vi "Add Stage Section.vi"(8 "error in (no error)":errorcluster, 10 "Analysis Options":T1={"Pull In Time"=TRUE, "Pull In Max Current"=TRUE, "Pull In Max Voltage"=TRUE, "Pull In Min Voltage"=TRUE, "Pull In Avg Voltage"=TRUE, "Hold In Time"=TRUE, "Hold In Max Current"=TRUE, "Hold In Min Current"=TRUE, "Hold In Avg Current"=TRUE, "Hold In Max Voltage"=TRUE, "Hold In Min Voltage"=TRUE, "Hold In Avg Max Voltage"=TRUE, "Hold In Avg Min Voltage"=TRUE, "Off Time"=TRUE, "Off Stage Max Current"=TRUE, "Off Stage Min Current"=TRUE, "Off Stage Avg Current"=TRUE, "Off Stage Max Voltage"=TRUE, "Off Stage Min Voltage"=TRUE, "Off Stage Avg Voltage"=TRUE, "Total Voltage Pulses"=TRUE, "Total Stage Time"=TRUE}, 11 "Shot Section reference in":T2=18446744073709551615 format="%.0x") -> (0 "error out":errorcluster, 3 "Shot Section reference out":T2=18446744073709551615 format="%.0x")   [LabVIEW 2015, in "Fuel Injector Analysis Addon System Explorer.lvlib"]
uses:
  Fuel Injector Analysis Addon System Explorer.lvlib
  <vilib>/NI Veristand/Custom Device API/Custom Device Item Ref.ctl
  Shared/Types/Analysis.Channels.Select.ctl
  <vilib>/NI Veristand/Custom Device API/Custom Device Channel.ctl
  <vilib>/NI Veristand/Custom Device API/Custom Device Channel Type.ctl
  Shared/Constants.vi
  Shared/Fuel Injector Analysis Addon Shared.lvlib
  <vilib>/NI Veristand/Custom Device API/Custom Device API.lvlib
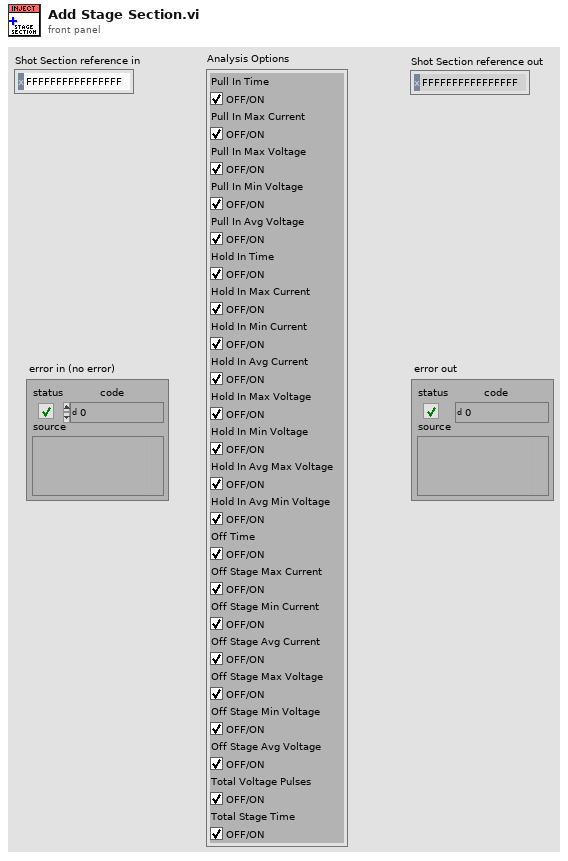
[diagram p1: front panel]
types:
  T1 = typedef "Fuel Injector Analysis Addon Shared.lvlib/Analysis.Channels.Select.ctl" = cluster{"Pull In Time":bool, "Pull In Max Current":bool, "Pull In Max Voltage":bool, "Pull In Min Voltage":bool, "Pull In Avg Voltage":bool, "Hold In Time":bool, "Hold In Max Current":bool, "Hold In Min Current":bool, "Hold In Avg Current":bool, "Hold In Max Voltage":bool, "Hold In Min Voltage":bool, "Hold In Avg Max Voltage":bool, "Hold In Avg Min Voltage":bool, "Off Time":bool, "Off Stage Max Current":bool, "Off Stage Min Current":bool, "Off Stage Avg Current":bool, "Off Stage Max Voltage":bool, "Off Stage Min Voltage":bool, "Off Stage Avg Voltage":bool, "Total Voltage Pulses":bool, "Total Stage Time":bool}
  T2 = typedef "Custom Device API.lvlib/Custom Device Item Ref.ctl" = u64
  T3 = typedef "Custom Device API.lvlib/Custom Device Channel.ctl" = cluster{"Type":T4, "Units":string, "Default Value":dbl, "Faultable":bool, "Scalable":bool}
  T4 = typedef "Custom Device API.lvlib/Custom Device Channel Type.ctl" = enum16{"Input", "Output"}
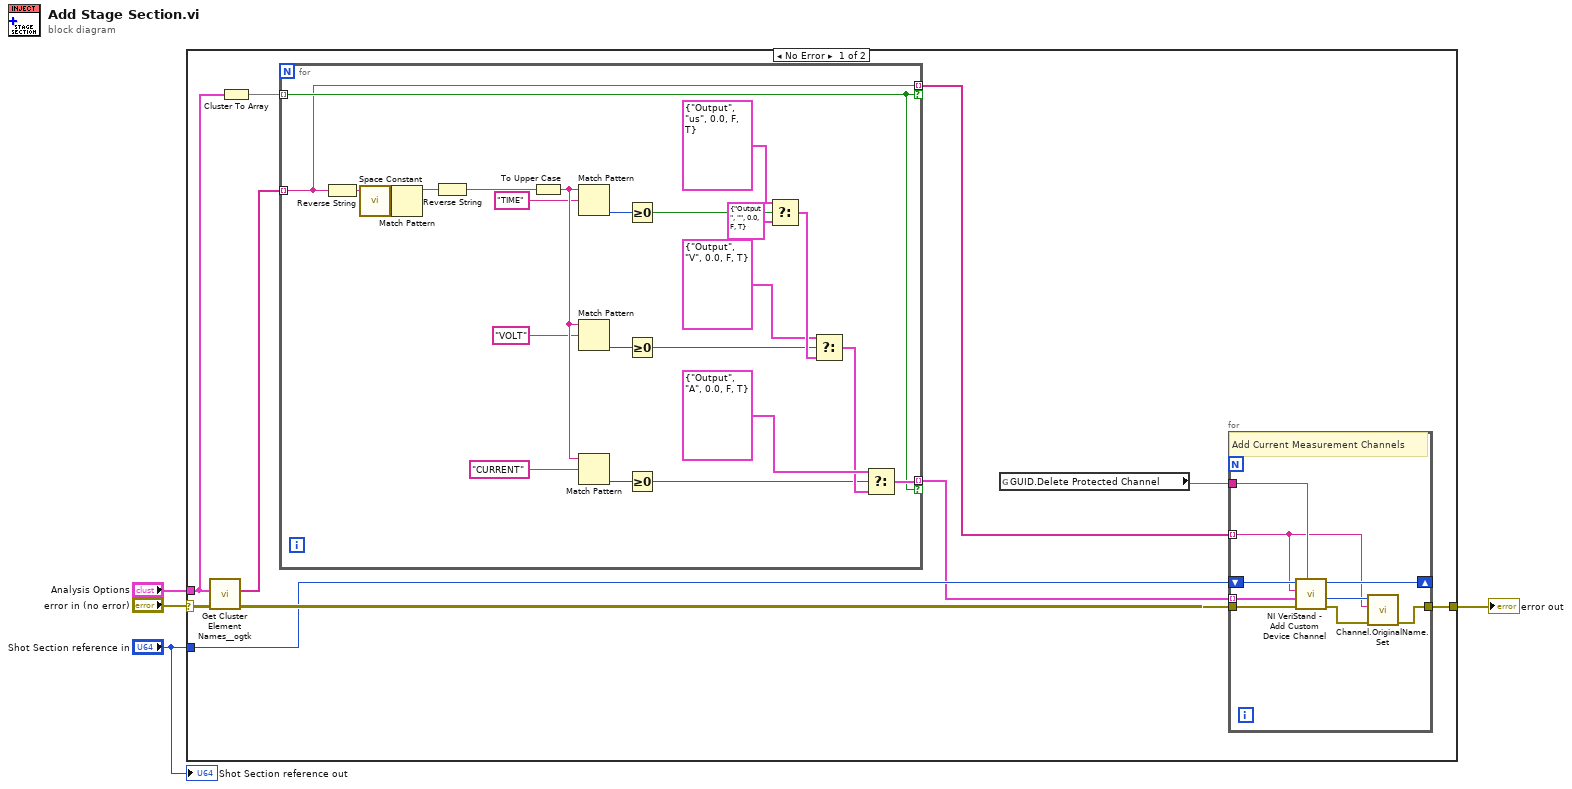
[diagram p0: block diagram]
diagram:
  n1 = case shown="No Error" "error in (no error)" {
    selector: "error in (no error)" -> [w12 w47]
    tunnel: "Shot Section reference in" -> [w13 _]
    tunnel: [w8 w47] -> w3
    tunnel: "Analysis Options" -> [w10 _]
    frame No Error {
      n2 = call <userlib>:"Get Cluster Element Names__ogtk.vi"("error in (no error)"=w12, "Cluster"=w10) -> ("error out"=w11:errorcluster, "Element Names"=w6:string[])  [unwired: 8 in]
      n3 = Cluster To Array(cluster=w10) -> (array=w9:bool[])
      n4 = for {
        tunnel: w6 -> [w19] mode=indexing
        tunnel: w9 -> [w23] mode=indexing
        tunnel: [w25] -> w7 mode=indexing if=w23
        tunnel: [w19] -> w5 mode=indexing if=w23
        n5 = Reverse String(1:w19) -> (0:w18:string)
        n6 = call <vilib>:"Space Constant.vi"() -> ("String"=w17:string)
        n7 = Match Pattern(string=w18, regular expression=w17) -> (before substring=w15:string)  [unwired: 1 in, 3 out]
        n8 = Reverse String(1:w15) -> (0:w16:string)
        n9 = To Upper Case(1:w16) -> (0:w37:string)
        n10 = Match Pattern(string=w37, regular expression="TIME") -> (offset past match=w33:i32)  [unwired: 1 in, 3 out]
        n11 = Match Pattern(string=w37, regular expression="VOLT") -> (offset past match=w32:i32)  [unwired: 1 in, 3 out]
        n12 = Match Pattern(string=w37, regular expression="CURRENT") -> (offset past match=w31:i32)  [unwired: 1 in, 3 out]
        n13 = Greater Or Equal To 0?(x=w33) -> (x >= 0?=w20:bool)
        n14 = Greater Or Equal To 0?(x=w32) -> (x >= 0?=w21:bool)
        n15 = Greater Or Equal To 0?(x=w31) -> (x >= 0?=w22:bool)
        n16 = Select(t=T3 {"Type"=enum."Output", "Units"="us", "Default Value"=0.0, "Faultable"=FALSE, "Scalable"=TRUE} ("Channel"), s=w20, f=T3 {"Type"=enum."Output", "Units"="", "Default Value"=0.0, "Faultable"=FALSE, "Scalable"=TRUE}) -> (s? t:f=w29:T3)
        n17 = Select(t=T3 {"Type"=enum."Output", "Units"="V", "Default Value"=0.0, "Faultable"=FALSE, "Scalable"=TRUE} ("Channel"), s=w21, f=w29) -> (s? t:f=w26:T3)
        n18 = Select(t=T3 {"Type"=enum."Output", "Units"="A", "Default Value"=0.0, "Faultable"=FALSE, "Scalable"=TRUE} ("Channel"), s=w22, f=w26) -> (s? t:f=w25:T3)
      }
      n19 = global read "Constants.vi" "GUID.Delete Protected Channel"() -> (w14:string)
      n20 = for {
        tunnel: w5 -> [w38] mode=indexing
        tunnel: w11 -> [w46]
        tunnel: w14 -> [w44]
        tunnel: [w39] -> w8
        shift-right: [w43] -> _
        shift-left: w13 -> [w45]
        tunnel: w7 -> [w42] mode=indexing
        # "Add Current Measurement Channels"
        n21 = call <vilib>:"NI VeriStand - Add Custom Device Channel.vi"("GUID (Default Channel)"=w44, "error in (no error)"=w46, "Channel"=w42, "Channel Name"=w38, "Parent Ref in"=w45) -> ("error out"=w40:errorcluster, "Channel Ref"=w41:T2, "Parent Ref out"=w43:T2)  [unwired: 3 in, 1 out]
        n22 = call "Channel.OriginalName.Set.vi"("error in (no error)"=w40, "Constants.Channel Name"=w38, "Ref"=w41) -> ("error out"=w39:errorcluster)  [unwired: 7 in, 1 out]
      }
    }
    frame Error {
    }
  }
  "error out" <- w3
  "Shot Section reference out" <- "Shot Section reference in"
